vi "Create bounding rectangle based on center.vi"(1 "x center":i16, 2 "y center":i16, 3 "distance from x/y center":i16) -> (0 "bounding rectangle coordinates":cluster{i16, i16, i16, i16})   [LabVIEW 2010]
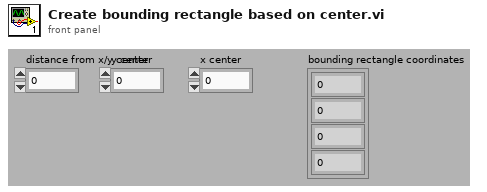
[diagram p1: front panel]
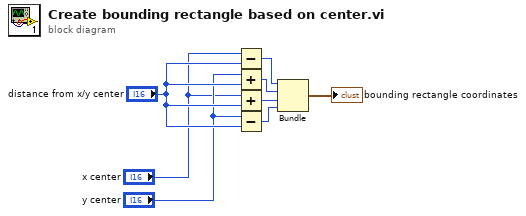
[diagram p0: block diagram]
diagram:
  n1 = Subtract(x="x center", y="distance from x/y center") -> (x-y=w4:i16)
  n2 = Add(x="y center", y="distance from x/y center") -> (x+y=w5:i16)
  n3 = Add(x="x center", y="distance from x/y center") -> (x+y=w6:i16)
  n4 = Subtract(x="y center", y="distance from x/y center") -> (x-y=w7:i16)
  n5 = Bundle(w4, w5, w6, w7) -> (→"bounding rectangle coordinates":cluster{i16, i16, i16, i16})  [unwired: 1 in]
